vi "2D Array.vi"() -> ()   [LabVIEW 2009]
panel:
  in  "Number of coloumns":dbl
  in  "Number of rows":dbl
  out "Array":dbl[][](array[numeric])
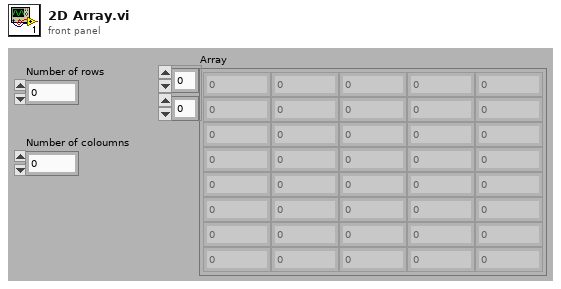
[diagram p1: front panel]
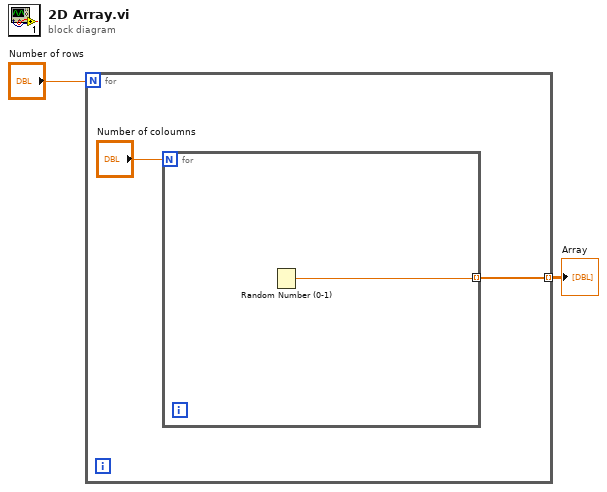
[diagram p0: block diagram]
diagram:
  n1 = for {
    N: "Number of rows" -> [_]
    tunnel: [w4] -> w2 mode=indexing
    n2 = for {
      N: "Number of coloumns" -> [_]
      tunnel: [w5] -> w4 mode=indexing
      n3 = Random Number (0-1)() -> (number: 0 to 1=w5:dbl)
    }
  }
  "Array" <- w2
